vi "GenSINEx2PtByPt.vi"(9 "Time":dbl format="%0.2f", 11 "Acción de Control":dbl) -> (1 "Fase Control":dbl, 3 "Fase Fija":dbl format="%0.2f")   [LabVIEW 2011, in "GripsMaster.lvclass"]
uses:
  GripsMaster.lvclass
  <vilib>/ptbypt/NI_PtbyPt.lvlib
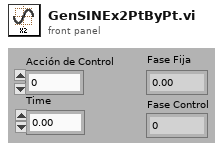
[diagram p1: front panel]
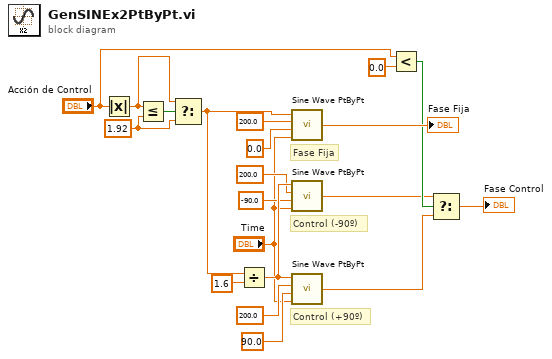
[diagram p0: block diagram]
diagram:
  w20 = 1.92 ("y")
  # "Control (+90º)"
  # "Control (-90º)"
  # "Fase Fija"
  n1 = Absolute Value(x="Acción de Control") -> (abs(x)=w8:dbl)
  n2 = Less Or Equal?(x=w8, y=w20) -> (x <= y?=w19:bool)
  n3 = Select(t=w8, s=w19, f=w20) -> (s? t:f=w2:dbl)
  n4 = Divide(x=w2, y=1.6) -> (x/y=w13:dbl)
  n5 = call <vilib>:"Sine Wave PtByPt.vi"("time"="Time", "phase"=0.0, "frequency"=200.0, "amplitude"=w2) -> ("sine wave"=→"Fase Fija":dbl)
  n6 = call <vilib>:"Sine Wave PtByPt.vi"("time"="Time", "phase"=-90.0, "frequency"=200.0, "amplitude"=w13) -> ("sine wave"=w5:dbl)
  n7 = call <vilib>:"Sine Wave PtByPt.vi"("time"="Time", "phase"=90.0, "frequency"=200.0, "amplitude"=w13) -> ("sine wave"=w4:dbl)
  n8 = Less?(x="Acción de Control", y=0.0) -> (x < y?=w6:bool)
  n9 = Select(t=w5, s=w6, f=w4) -> (s? t:f=→"Fase Control":dbl)
